vi "LAChatByUserTask.vi"(8 "Error In":errorcluster, 10 "UserTask":T1, 11 "LiteAgent In":T2) -> (0 "Error Out":errorcluster, 3 "LiteAgent Out":T2)   [LabVIEW 2017, in "LiteAgentSDK.lvlib"]
uses:
  LiteAgentSDK.lvlib
  C:/Users/Jan/Projects/LiteAgentSDK-LabVIEW/Source/Bin/LiteAgentSDK.LabVIEW.dll
  Bin/LiteAgentSDK.LabVIEW.dll
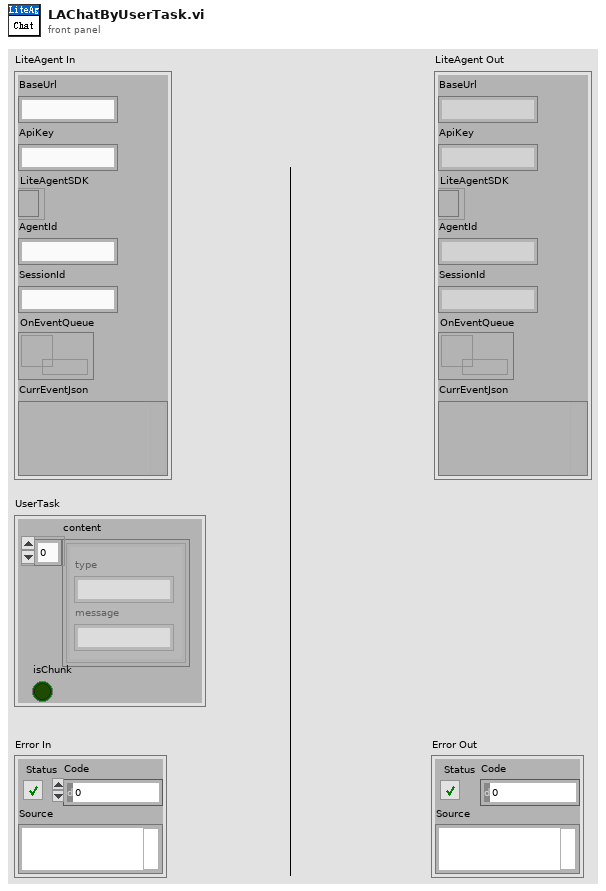
[diagram p1: front panel]
types:
  T1 = cluster{"content":cluster{"type":string, "message":string}[], "isChunk":bool}
  T2 = cluster{"BaseUrl":string, "ApiKey":string, "LiteAgentSDK":refnum<k24>, "AgentId":string, "SessionId":string, "OnEventQueue":refnum<queue>, "CurrEventJson":variant}
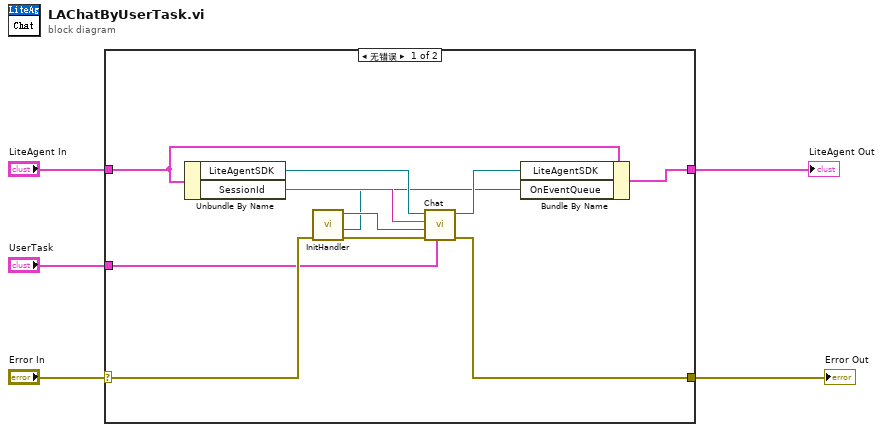
[diagram p0: block diagram]
diagram:
  n1 = case shown="无错误" "Error In" {
    selector: "Error In" -> [w16 w18]
    tunnel: [w14 w18] -> w4
    tunnel: "LiteAgent In" -> [w6 w17]
    tunnel: [w7 w17] -> w2
    tunnel: "UserTask" -> [w10 _]
    frame No Error {
      n2 = Unbundle By Name(w6) -> ("LiteAgentSDK"=w12:refnum<k24>, "SessionId"=w11:string)
      n3 = call "InitHandler.vi"("Error Input"=w16) -> ("Error Output"=w15:errorcluster, "Queue Out"=w8:refnum<queue>, "AgentMessageEventHandler"=w13:refnum<k24>)  [unwired: 8 in]
      n4 = call "Chat.vi"("UserTask"=w10, "Error Input"=w15, "AgentMessageEventHandler"=w13, "SessionId"=w11, "LiteAgentSDK Input"=w12) -> ("Error Output"=w14:errorcluster, "LiteAgentSDK Output"=w9:refnum<k24>)  [unwired: 5 in]
      n5 = Bundle By Name(cluster=w6, "LiteAgentSDK"=w9, "OnEventQueue"=w8) -> (w7:T2)
    }
    frame Error {
    }
  }
  "Error Out" <- w4
  "LiteAgent Out" <- w2
